vi "Get Summary Variables.vi"(8 "error in (no error)":errorcluster, 10 "Mute":i32, 11 "LabVIEW Web Service Request":refnum<class "Web Request.lvclass">) -> (0 "error out":errorcluster, 3 "LabVIEW Web Service Request out":refnum<class "Web Request.lvclass">)   [LabVIEW 2018]
doc: "This VI sets all of the ESP variables for a single contact so it can be output from an ESP script."
uses:
  <vilib>/wsapi/Web Request.lvclass
  channel_cluster.ctl
  CAEN globals.vi
  subvis/i32 to dec string small.vi
  subvis/dbl to fr string small.vi
  subvis/bool to string small.vi
  <vilib>/wsapi/class/subVIs/Set Many String ESP Variables.vi
panel:
  out "result string":string
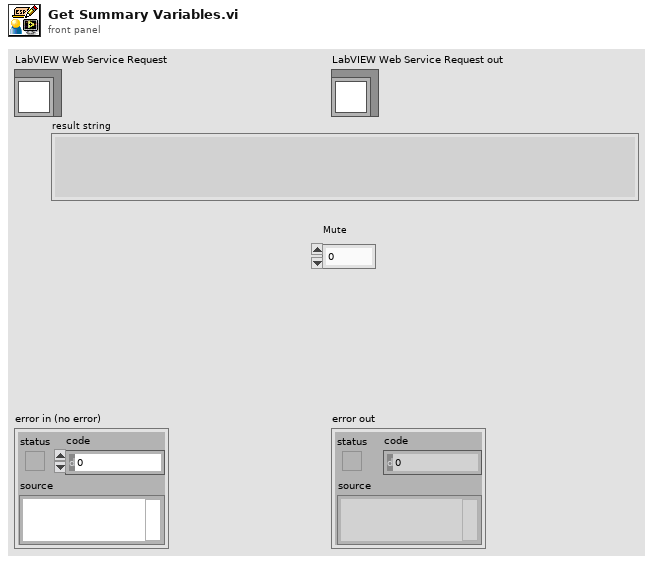
[diagram p1: front panel]
types:
  T1 = typedef "channel_cluster.ctl" = cluster{"Channel Name":string, "Crate":i32, "Card Type":string, "Card":i32, "Channel":i32, "Status Icon":picture, "Vmon (V)":dbl, "Vset (V)":dbl, "Imon (A)":dbl, "Iset (A)":dbl, "Timestamp":string, "ON/OFF":bool, "Status":string, "Vswmax (V)":dbl, "Flag":bool, "Vfile (V)":dbl, "Error Logged":bool[], "enable_file":bool}
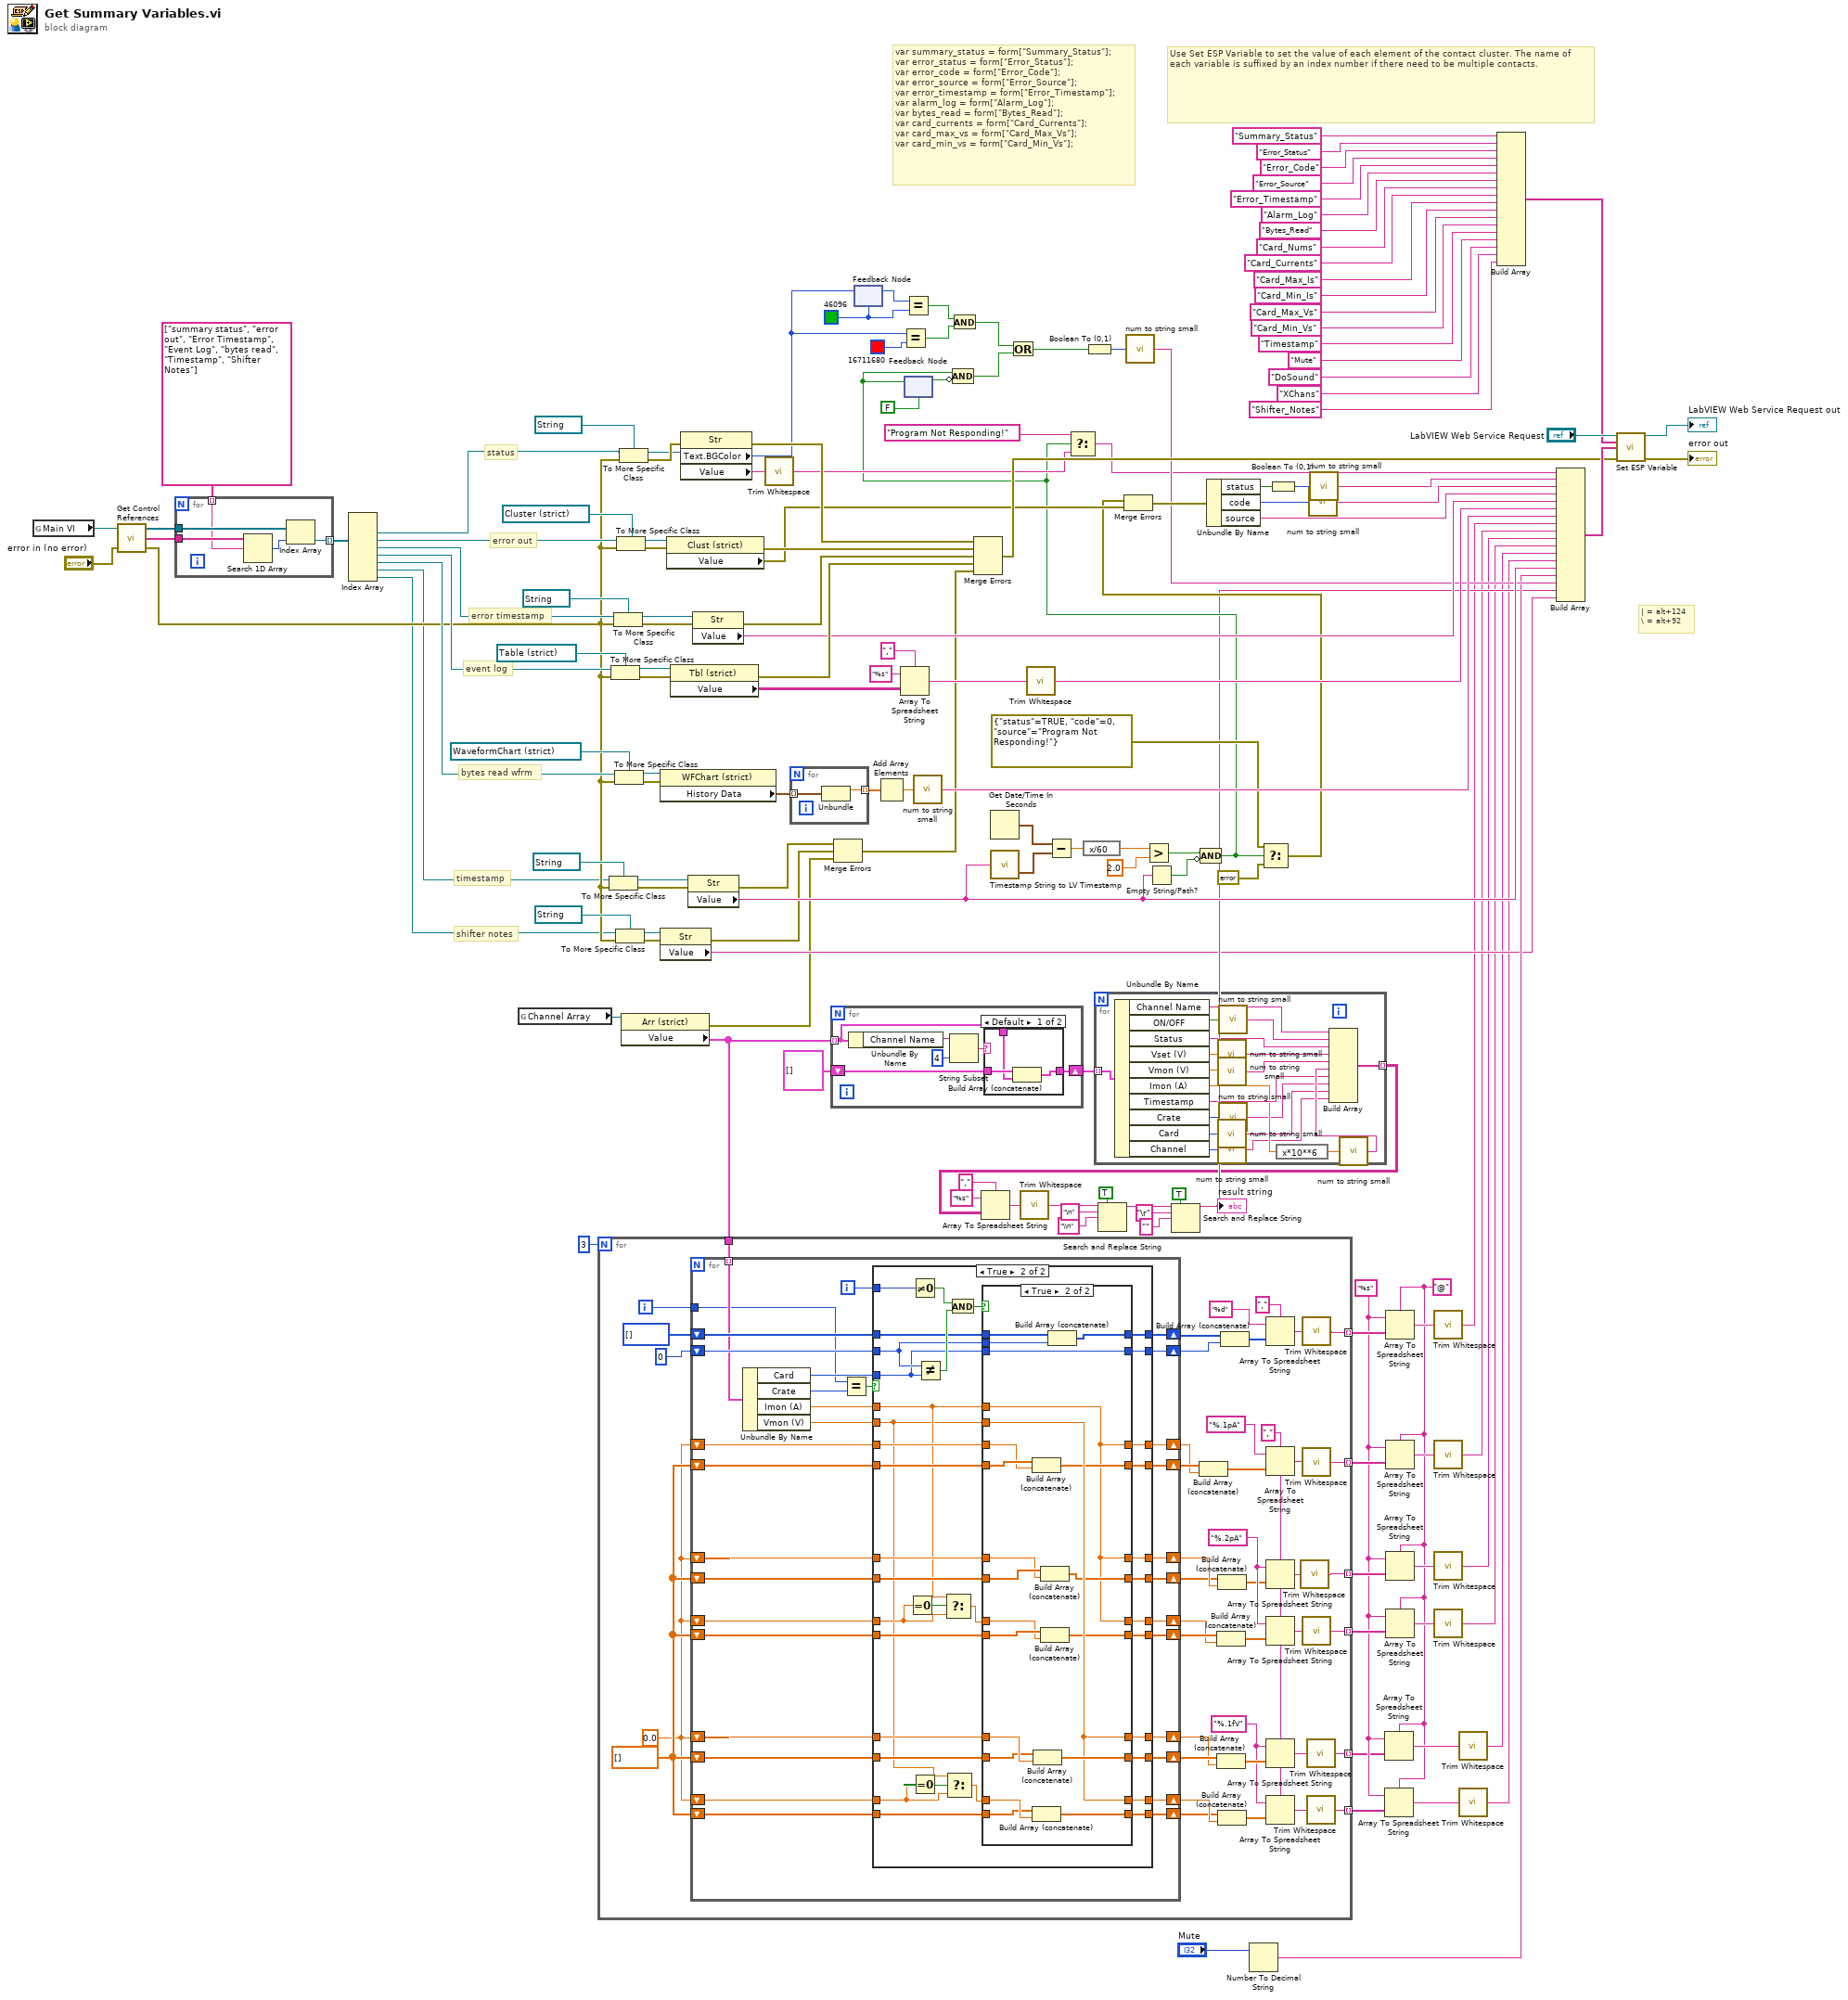
[diagram p0: block diagram]
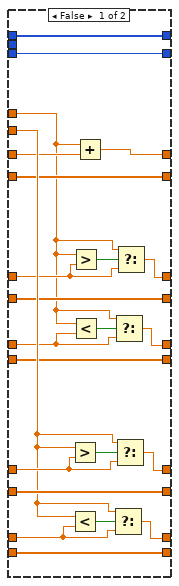
[diagram p3: hidden frame]
diagram:
  w4 = "@" ("delimiter (Tab)")
  w3 = "%s" ("format string")
  w68 = u32 46096
  # "shifter notes"
  # "timestamp"
  # "bytes read wfrm"
  # "event log"
  # "error timestamp"
  # "error out"
  # "status"
  # "| = alt+124\n\\ = alt+92"
  # "var summary_status = form[\"Summary_Status\"];\nvar error_status = form[\"Error_Status\"];\nvar error_code = form[\"Error_Code\"];\nvar error_source = form[\"Error_Source\"];\nvar error_timestamp = form[\"Error_Timestamp\"];\nvar alarm_log = form[\"Alarm_Log\"];\nvar bytes_read = form[\"Bytes_Read\"];\nvar card_currents = form[\"Card_Currents\"];\nvar card_max_vs = form[\"Card_Max_Vs\"];\nvar card_min_vs = form[\"Card_Min_Vs\"];"
  # "Use Set ESP Variable to set the value of each element of the contact cluster. The name of each variable is suffixed by an index number if there need to be multiple contacts."
  n1 = global read "CAEN globals.vi" "Main VI"() -> (w144:refnum<vi>)
  n2 = call "Get Control References.vi"("error in"="error in (no error)", "This vi"=w144) -> ("error out"=w25:errorcluster, "Control Names"=w143:string[], "Controls[]"=w142:refnum<vi>[])  [unwired: 1 in]
  n3 = for {
    tunnel: w143 -> [w160]
    tunnel: w142 -> [w158]
    tunnel: [w157] -> w135 mode=indexing
    tunnel: string[] ["summary status", "error out", "Error Timestamp", "Event Log", "bytes read", "Timestamp", "Shifter Notes"] ("Control Names") -> [w156] mode=indexing
    n4 = Search 1D Array(1D array=w160, element=w156) -> (index of element=w159:i32)  [unwired: 1 in]
    n5 = Index Array(array=w158, index=w159) -> (element=w157:refnum<vi>)
  }
  n6 = Index Array(array=w135) -> (element #1=w133:refnum<vi>, element #2=w130:refnum<vi>, element #3=w127:refnum<vi>, element #4=w120:refnum<vi>, element #5=w119:refnum<vi>, element #6=w24:refnum<vi>, element #7=w23:refnum<vi>)  [unwired: 7 in]
  n7 = global read "CAEN globals.vi" "Channel Array"() -> (w28:refnum<vi>)
  n8 = To More Specific Class(target class=refnum<vi> refnum ("Label.Text"), reference=w24, error in=w25) -> (specific class reference=w89:refnum<vi>, error out=w88:errorcluster)
  n9 = To More Specific Class(target class=refnum<vi> refnum ("Alarm Log"), reference=w120, error in=w25) -> (specific class reference=w122:refnum<vi>, error out=w121:errorcluster)
  n10 = To More Specific Class(target class=refnum<vi> refnum ("Label.Text"), reference=w127, error in=w25) -> (specific class reference=w125:refnum<vi>, error out=w126:errorcluster)
  n11 = To More Specific Class(target class=refnum<vi> refnum ("bytes read 2"), reference=w119, error in=w25) -> (specific class reference=w123:refnum<vi>, error out=w124:errorcluster)
  n12 = To More Specific Class(target class=refnum<vi> refnum ("Label.Text"), reference=w23, error in=w25) -> (specific class reference=w35:refnum<vi>, error out=w34:errorcluster)
  n13 = To More Specific Class(target class=refnum<vi> refnum ("error in (no error)"), reference=w130, error in=w25) -> (specific class reference=w129:refnum<vi>, error out=w131:errorcluster)
  n14 = To More Specific Class(target class=refnum<vi> refnum ("Label.Text"), reference=w133, error in=w25) -> (specific class reference=w132:refnum<vi>, error out=w134:errorcluster)
  n15 = property class="Arr (strict)"(reference=w28) -> (error out=w26:errorcluster, "Value"=w22:T1[])  [unwired: 1 in, 1 out]
  n16 = for {
    N: 3 -> [_]
    tunnel: [w169] -> w10 mode=indexing
    tunnel: [w171] -> w7 mode=indexing
    tunnel: [w167] -> w8 mode=indexing
    tunnel: [w165] -> w9 mode=indexing
    tunnel: w22 -> [w176]
    tunnel: [w163] -> w1 mode=indexing
    tunnel: [w161] -> w2 mode=indexing
    i -> [w173]
    w184 = "%.2pA" ("format string")
    w177 = "," ("delimiter (Tab)")
    w193 = "%.1fV" ("format string")
    w175 = dbl[] []
    w174 = 0.0 ("ReadBufferView")
    n17 = for {
      shift-right: [w231] -> w199
      shift-left: w174 -> [w234]
      shift-right: [w220] -> w186
      shift-left: 0 ("Card") -> [w219]
      shift-right: [w233] -> w200
      shift-left: w175 -> [w232]
      shift-right: [w229] -> w201
      shift-left: w175 -> [w230]
      shift-right: [w228] -> w202
      shift-left: w174 -> [w218]
      shift-right: [w224] -> w198
      shift-left: w175 -> [w225]
      shift-right: [w226] -> w197
      shift-left: w174 -> [w227]
      shift-right: [w221] -> w187
      shift-left: i32[] [] ("appended array") -> [w222]
      shift-right: [w213] -> w181
      shift-left: w174 -> [w210]
      shift-right: [w211] -> w180
      shift-left: w175 -> [w212]
      shift-right: [w215] -> w179
      shift-left: w175 -> [w214]
      shift-right: [w216] -> w178
      shift-left: w174 -> [w217]
      tunnel: w176 -> [w208] mode=indexing
      tunnel: w173 -> [w203]
      i -> [w223]
      n18 = Unbundle By Name(w208) -> ("Card"=w206:i32, "Crate"=w204:i32, "Imon (A)"=w209:dbl, "Vmon (V)"=w207:dbl)
      n19 = Equal?(x=w203, y=w204) -> (x = y?=w205:bool)
      n20 = case shown="True" w205 {
        tunnel: w234 -> [w238 w281]
        tunnel: [w237 w280] -> w233
        tunnel: w232 -> [w237 w279]
        tunnel: [w238 w278] -> w231
        tunnel: w230 -> [w235 w277]
        tunnel: [w235 w276] -> w229
        tunnel: [w236 w275] -> w228
        tunnel: w227 -> [w244 w274]
        tunnel: [w244 w273] -> w226
        tunnel: w225 -> [w243 w272]
        tunnel: [w243 w271] -> w224
        tunnel: w223 -> [_ w268]
        tunnel: w222 -> [w246 w266]
        tunnel: [w246 w265] -> w221
        tunnel: [w245 w264] -> w220
        tunnel: w219 -> [w245 w263]
        tunnel: w218 -> [w236 w261]
        tunnel: w217 -> [w240 w258]
        tunnel: [w240 w256] -> w216
        tunnel: [w239 w255] -> w215
        tunnel: w214 -> [w239 w254]
        tunnel: [w242 w253] -> w213
        tunnel: w212 -> [w241 w252]
        tunnel: [w241 w251] -> w211
        tunnel: w210 -> [w242 w250]
        tunnel: w209 -> [_ w249]
        tunnel: w207 -> [_ w248]
        tunnel: w206 -> [_ w247]
        frame False {
        }
        frame True {
          n21 = Equal To 0?(x=w258) -> (x = 0?=w257:bool)
          n22 = Not Equal To 0?(x=w268) -> (x != 0?=w267:bool)
          n23 = Equal To 0?(x=w261) -> (x = 0?=w262:bool)
          n24 = Not Equal?(x=w263, y=w247) -> (x != y?=w270:bool)
          n25 = Select(t=w249, s=w257, f=w258) -> (s? t:f=w259:dbl)
          n26 = Select(t=w248, s=w262, f=w261) -> (s? t:f=w260:dbl)
          n27 = And(x=w267, y=w270) -> (x .and. y?=w269:bool)
          n28 = case shown="True" w269 {
            tunnel: w281 -> [w303 w325]
            tunnel: [w304 w324] -> w280
            tunnel: w279 -> [w304 w323]
            tunnel: w248 -> [w299 w319]
            tunnel: [w301 w319] -> w278
            tunnel: w277 -> [w298 w321]
            tunnel: w260 -> [w296 w322]
            tunnel: [w298 w320] -> w276
            tunnel: [w297 w319] -> w275
            tunnel: w274 -> [w295 w316]
            tunnel: w249 -> [w282 w308]
            tunnel: [w294 w308] -> w273
            tunnel: w272 -> [w293 w318]
            tunnel: [w293 w317] -> w271
            tunnel: w247 -> [w291 w313]
            tunnel: w266 -> [w292 w315]
            tunnel: [w292 w314] -> w265
            tunnel: [w291 w313] -> w264
            tunnel: w263 -> [_ w312]
            tunnel: w250 -> [w284 w310]
            tunnel: [w283 w309] -> w251
            tunnel: w252 -> [w283 w311]
            tunnel: [w286 w308] -> w253
            tunnel: w254 -> [w288 w307]
            tunnel: w259 -> [w290 w305]
            tunnel: [w288 w306] -> w255
            tunnel: [w289 w308] -> w256
            frame False {
              n29 = Greater?(x=w299, y=w303) -> (0:w302:bool)
              n30 = Less?(x=w299, y=w296) -> (x < y?=w300:bool)
              n31 = Greater?(x=w282, y=w284) -> (0:w285:bool)
              n32 = Less?(x=w282, y=w290) -> (x < y?=w287:bool)
              n33 = Add(x=w282, y=w295) -> (x+y=w294:dbl)
              n34 = Select(t=w299, s=w300, f=w296) -> (s? t:f=w297:dbl)
              n35 = Select(t=w282, s=w287, f=w290) -> (s? t:f=w289:dbl)
              n36 = Select(t=w299, s=w302, f=w303) -> (s? t:f=w301:dbl)
              n37 = Select(t=w282, s=w285, f=w284) -> (s? t:f=w286:dbl)
            }
            frame True {
              n38 = Build Array (concatenate)(w318, w316) -> (w317:dbl[])
              n39 = Build Array (concatenate)(w321, w322) -> (w320:dbl[])
              n40 = Build Array (concatenate)(w323, w325) -> (w324:dbl[])
              n41 = Build Array (concatenate)(w311, w310) -> (w309:dbl[])
              n42 = Build Array (concatenate)(w307, w305) -> (w306:dbl[])
              n43 = Build Array (concatenate)(w315, w312) -> (w314:i32[])
            }
          }
        }
      }
    }
    n44 = Build Array (concatenate)(w198, w197) -> (w196:dbl[])
    n45 = Build Array (concatenate)(w179, w178) -> (w182:dbl[])
    n46 = Build Array (concatenate)(w200, w199) -> (w194:dbl[])
    n47 = Build Array (concatenate)(w180, w181) -> (w183:dbl[])
    n48 = Build Array (concatenate)(w201, w202) -> (w195:dbl[])
    n49 = Build Array (concatenate)(w187, w186) -> (w188:i32[])
    n50 = Array To Spreadsheet String(delimiter (Tab)=",", array=w188, 3:"%d" ("format string")) -> (spreadsheet string=w172:string)
    n51 = Array To Spreadsheet String(delimiter (Tab)=w177, array=w196, 3:"%.1pA" ("format string")) -> (spreadsheet string=w170:string)
    n52 = Array To Spreadsheet String(delimiter (Tab)=w177, array=w183, 3:w184) -> (spreadsheet string=w168:string)
    n53 = Array To Spreadsheet String(delimiter (Tab)=w177, array=w182, 3:w184) -> (spreadsheet string=w166:string)
    n54 = Array To Spreadsheet String(delimiter (Tab)=w177, array=w194, 3:w193) -> (spreadsheet string=w164:string)
    n55 = Array To Spreadsheet String(delimiter (Tab)=w177, array=w195, 3:w193) -> (spreadsheet string=w162:string)
    n56 = call <vilib>:"Trim Whitespace.vi"("string"=w168) -> ("trimmed string"=w167:string)  [unwired: 1 in]
    n57 = call <vilib>:"Trim Whitespace.vi"("string"=w172) -> ("trimmed string"=w171:string)  [unwired: 1 in]
    n58 = call <vilib>:"Trim Whitespace.vi"("string"=w170) -> ("trimmed string"=w169:string)  [unwired: 1 in]
    n59 = call <vilib>:"Trim Whitespace.vi"("string"=w166) -> ("trimmed string"=w165:string)  [unwired: 1 in]
    n60 = call <vilib>:"Trim Whitespace.vi"("string"=w164) -> ("trimmed string"=w163:string)  [unwired: 1 in]
    n61 = call <vilib>:"Trim Whitespace.vi"("string"=w162) -> ("trimmed string"=w161:string)  [unwired: 1 in]
  }
  n62 = property class="WFChart (strict)"(reference=w123, error in=w124) -> ("History Data"=w100:cluster{dbl, "element":i32}[])  [unwired: 2 out]
  n63 = property class="Str"(reference=w35, error in=w34) -> (error out=w27:errorcluster, "Value"=w33:string)  [unwired: 1 out]
  n64 = property class="Clust (strict)"(reference=w129, error in=w131) -> (error out=w116:errorcluster, "Value"=w87:errorcluster)  [unwired: 1 out]
  n65 = property class="Tbl (strict)"(reference=w122, error in=w121) -> (error out=w114:errorcluster, "Value"=w104:string[][])  [unwired: 1 out]
  n66 = property class="Str"(reference=w132, error in=w134) -> (error out=w117:errorcluster, "Text.BGColor"=w71:u32, "Value"=w74:string)  [unwired: 1 out]
  n67 = property class="Str"(reference=w89, error in=w88) -> (error out=w55:errorcluster, "Value"=w78:string)  [unwired: 1 out]
  n68 = property class="Str"(reference=w125, error in=w126) -> (error out=w115:errorcluster, "Value"=w106:string)  [unwired: 1 out]
  n69 = call <vilib>:"Trim Whitespace.vi"("string"=w74) -> ("trimmed string"=w44:string)  [unwired: 1 in]
  n70 = for {
    tunnel: w100 -> [w327] mode=indexing
    tunnel: [w326] -> w99 mode=indexing
    n71 = Unbundle(w327) -> (w326:dbl)  [unwired: 1 out]
  }
  n72 = for {
    tunnel: w22 -> [w328] mode=indexing
    shift-right: [w330] -> w30
    shift-left: T1[] [] -> [w329]
    n73 = Unbundle By Name(w328) -> ("Channel Name"=w333:string)
    n74 = String Subset(string=w333, length (rest)=4 ("length (rest)")) -> (substring=w331:string)  [unwired: 1 in]
    n75 = case shown="Default" w331 {
      tunnel: [w336 w337] -> w330
      tunnel: w329 -> [w335 w337]
      tunnel: w328 -> [w334 _]
      frame Default {
        n76 = Build Array (concatenate)(w335, w334) -> (w336:T1[])
      }
      frame "CARD", "MRD_", "TNK_", "VETO" {
      }
    }
  }
  n77 = Merge Errors(w55, w27, w26) -> (w54:errorcluster)
  n78 = feedback-in #1(w71) -> ()
  n79 = feedback #1(w68) -> (w69:u32)
  n80 = Add Array Elements(numeric array=w99) -> (sum=w98:dbl)
  n81 = Array To Spreadsheet String(delimiter (Tab)=",", array=w104, 3:"%s" ("format string")) -> (spreadsheet string=w102:string)
  n82 = Equal?(x=w71, y=u32 16711680) -> (x = y?=w66:bool)
  n83 = Equal?(x=w69, y=w68) -> (x = y?=w67:bool)
  n84 = feedback #2(FALSE ("status")) -> (w59:bool)
  n85 = call-poly "num to string small.vi"("number"=w98) -> ("String"=w118:string)  [unwired: 14 in]
  n86 = And(x=w67, y=w66) -> (x .and. y?=w58:bool)
  n87 = Merge Errors(w117, w116, w115, w114, w54) -> (w113:errorcluster)
  n88 = Get Date/Time In Seconds() -> (seconds since 1Jan1904=w85:timestamp)
  n89 = call "Timestamp String to LV Timestamp.vi"("Timestamp String"=w78) -> ("Timestamp"=w84:timestamp)  [unwired: 1 out]
  n90 = call <vilib>:"Trim Whitespace.vi"("string"=w102) -> ("trimmed string"=w101:string)  [unwired: 1 in]
  n91 = Subtract(x=w85, y=w84) -> (x-y=w83:dbl)
  n92 = expression code="x/60"(w83) -> (w82:dbl)
  n93 = for {
    tunnel: w30 -> [w357] mode=indexing
    tunnel: [w346] -> w29 mode=indexing
    n94 = Unbundle By Name(w357) -> ("Channel Name"=w347:string, "ON/OFF"=w354:bool, "Status"=w349:string, "Vset (V)"=w355:dbl, "Vmon (V)"=w356:dbl, "Imon (A)"=w345:dbl, "Timestamp"=w350:string, "Crate"=w339:i32, "Card"=w342:i32, "Channel"=w343:i32)
    n95 = call-poly "num to string small.vi"("number"=w355) -> ("String"=w353:string)  [unwired: 14 in]
    n96 = call-poly "num to string small.vi"("number"=w356) -> ("String"=w352:string)  [unwired: 14 in]
    n97 = call-poly "num to string small.vi"("number"=w342) -> ("String"=w341:string)  [unwired: 14 in]
    n98 = call-poly "num to string small.vi"("number"=w343) -> ("String"=w340:string)  [unwired: 14 in]
    n99 = call-poly "num to string small.vi"("number"=w354) -> ("String"=w348:string)  [unwired: 14 in]
    n100 = call-poly "num to string small.vi"("number"=w339) -> ("String"=w338:string)  [unwired: 14 in]
    n101 = expression code="x*10**6"(w345) -> (w344:dbl)
    n102 = call-poly "num to string small.vi"("number"=w344) -> ("String"=w351:string)  [unwired: 14 in]
    n103 = Build Array(w347, w348, w349, w353, w352, w351, w350, w338, w341, w340) -> (w346:string[])
  }
  n104 = Array To Spreadsheet String(delimiter (Tab)=",", array=w29, 3:"%s" ("format string")) -> (spreadsheet string=w53:string)
  n105 = call <vilib>:"Trim Whitespace.vi"("string"=w53) -> ("trimmed string"=w46:string)  [unwired: 1 in]
  n106 = Search and Replace String(replace all?=TRUE ("replace all? (F)"), input string=w46, search string="\n", replace string="\\n" ("search string")) -> (result string=w38:string)  [unwired: 4 in, 3 out]
  n107 = Greater?(x=w82, y=2.0) -> (0:w77:bool)
  n108 = Empty String/Path?(string/path=w78) -> (empty?=w76:bool)
  n109 = Search and Replace String(replace all?=TRUE ("replace all? (F)"), input string=w38, search string="\r", replace string="" ("search string")) -> (result string=w37:string)  [unwired: 4 in, 3 out]
  "result string" <- w37
  n110 = Compound Arithmetic op=AND(w77, invert w76) -> (w42:bool)
  n111 = feedback-in #2(w42) -> ()
  n112 = Compound Arithmetic op=AND(w42, invert w59) -> (w57:bool)
  n113 = Or(x=w58, y=w57) -> (x .or. y?=w56:bool)
  n114 = Select(t="Program Not Responding!" ("source"), s=w42, f=w44) -> (s? t:f=w43:string)
  n115 = Boolean To (0,1)(Boolean=w56) -> (0, 1=w65:i16)
  n116 = call-poly "num to string small.vi"("number"=w65) -> ("String"=w64:string)  [unwired: 14 in]
  n117 = Number To Decimal String(number="Mute") -> (decimal integer string=w62:string)  [unwired: 1 in]
  n118 = Select(t=errorcluster {"status"=TRUE, "code"=0, "source"="Program Not Responding!"} ("error out"), s=w42, f=errorcluster {"status"=FALSE, "code"=0, "source"=""} ("error out")) -> (s? t:f=w61:errorcluster)
  n119 = Merge Errors(w61, w87) -> (w86:errorcluster)
  n120 = Unbundle By Name(w86) -> ("status"=w141:bool, "code"=w136:i32, "source"=w75:string)
  n121 = Boolean To (0,1)(Boolean=w141) -> (0, 1=w152:i16)
  n122 = call-poly "num to string small.vi"("number"=w136) -> ("String"=w137:string)  [unwired: 14 in]
  n123 = call-poly "num to string small.vi"("number"=w152) -> ("String"=w140:string)  [unwired: 14 in]
  n124 = Array To Spreadsheet String(delimiter (Tab)=w4, array=w1, 3:w3) -> (spreadsheet string=w6:string)
  n125 = Array To Spreadsheet String(delimiter (Tab)=w4, array=w2, 3:w3) -> (spreadsheet string=w5:string)
  n126 = Array To Spreadsheet String(delimiter (Tab)=w4, array=w7, 3:w3) -> (spreadsheet string=w20:string)
  n127 = Array To Spreadsheet String(delimiter (Tab)=w4, array=w10, 3:w3) -> (spreadsheet string=w12:string)
  n128 = Array To Spreadsheet String(delimiter (Tab)=w4, array=w8, 3:w3) -> (spreadsheet string=w14:string)
  n129 = Array To Spreadsheet String(delimiter (Tab)=w4, array=w9, 3:w3) -> (spreadsheet string=w16:string)
  n130 = call <vilib>:"Trim Whitespace.vi"("string"=w20) -> ("trimmed string"=w19:string)  [unwired: 1 in]
  n131 = call <vilib>:"Trim Whitespace.vi"("string"=w12) -> ("trimmed string"=w11:string)  [unwired: 1 in]
  n132 = call <vilib>:"Trim Whitespace.vi"("string"=w14) -> ("trimmed string"=w13:string)  [unwired: 1 in]
  n133 = call <vilib>:"Trim Whitespace.vi"("string"=w16) -> ("trimmed string"=w15:string)  [unwired: 1 in]
  n134 = call <vilib>:"Trim Whitespace.vi"("string"=w6) -> ("trimmed string"=w17:string)  [unwired: 1 in]
  n135 = call <vilib>:"Trim Whitespace.vi"("string"=w5) -> ("trimmed string"=w18:string)  [unwired: 1 in]
  n136 = Build Array("Summary_Status" ("string"), "Error_Status" ("string"), "Error_Code" ("string"), "Error_Source" ("string"), "Error_Timestamp" ("string"), "Alarm_Log" ("string"), "Bytes_Read" ("string"), "Card_Nums" ("string"), "Card_Currents" ("string"), "Card_Max_Is" ("string"), "Card_Min_Is" ("string"), "Card_Max_Vs" ("string"), "Card_Min_Vs" ("string"), "Timestamp" ("string"), "Mute" ("string"), "DoSound" ("string"), "XChans" ("string"), "Shifter_Notes" ("string")) -> (w154:string[])
  n137 = Build Array(w43, w140, w137, w75, w106, w101, w118, w19, w11, w13, w15, w17, w18, w78, w62, w64, w37, w33) -> (w153:string[])
  n138 = call-poly <vilib>:"Set ESP Variable.vi"("LabVIEW Web Service Request"="LabVIEW Web Service Request", "keys"=w154, "values"=w153, "error in (no error)"=w113) -> ("LabVIEW Web Service Request out"=→"LabVIEW Web Service Request out":refnum<class "Web Request.lvclass">, "error out"=→"error out":errorcluster)  [unwired: 10 in]
